vi "卫星模拟器自动控制软件.vi"() -> ()   [LabVIEW 2012]
uses:
  <vilib>/Utility/error.llb/DialogType.ctl
  <vilib>/DAQmx/create/channels.llb/DAQmx Create Channel (DO-Digital Output).vi
  <vilib>/vision/NI_Vision_Development_Module.lvlib
panel:
  in  "缩放比例 (像素/cm)":dbl=4.099468
  in  "远程数据记录器传输状态":bool
  in  "是否下传定位点信息":bool
  in  "远程端口":u16=61557
  in  "本地端口":u16=61556
  in  "远程终端地址":string="localhost"
  in  "broadcast":bool
  in  "是否姿态保持":bool
  out "alpha":dbl
  out "定位点信息":T1(array[cluster]) {"Aspect Ratio" format="%.2f"; "Orientation" format="%.2f"; "Area" format="%.2f"; "Object Center"."Y" format="%.2f"; "Object Center"."X" format="%.2f"}
  in  "Y中心校正":dbl
  in  "X中心校正":dbl
  out "相对偏角(deg)":dbl
  in  "目标Y":dbl
  in  "目标X":dbl
  out "X速率(cm/s)":dbl
  out "Y速率(cm/s)":dbl
  in  "OK Button":bool
  out "角速度(deg/s)":dbl
  in  "气浮状态":bool
  in  "控制频率(Hz)":u32=20
  in  "目标偏角":dbl
  in  "STOP":bool caption="stop (F)"
  out "导航相机输出":T2(plugin-control)
  out "alpha (deg)":dbl
  out "X偏移量 (cm)":dbl
  out "Y偏移量 (cm)":dbl
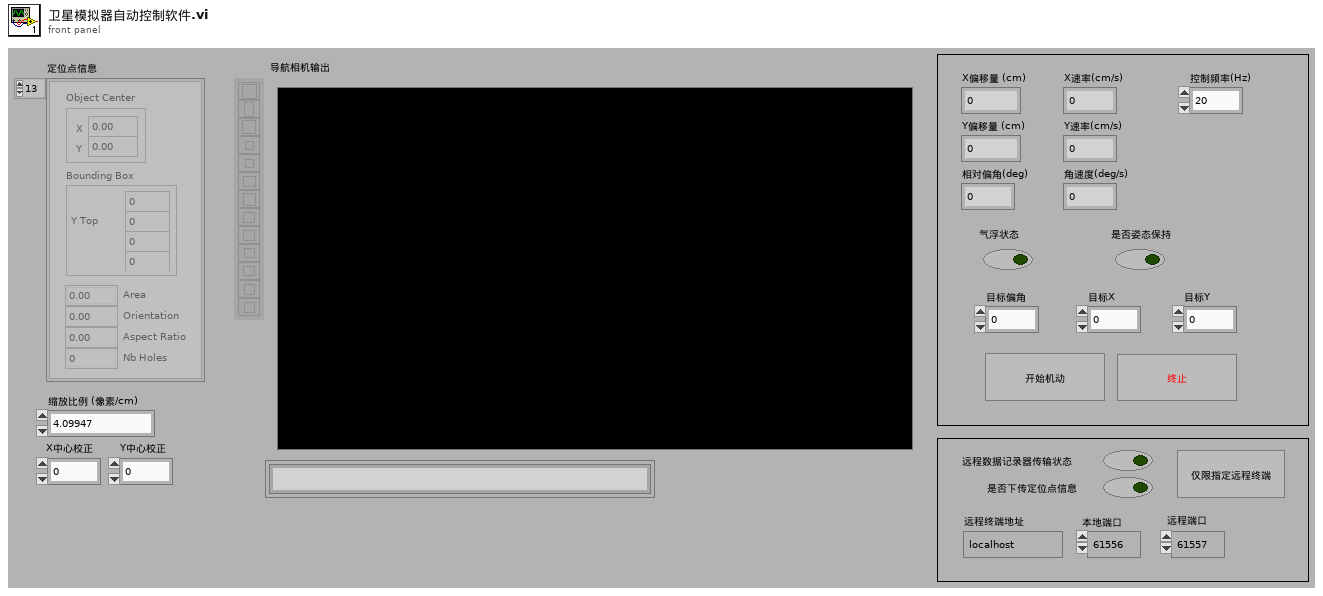
[diagram p1: front panel]
types:
  T1 = cluster{"Object Center":cluster{"X":sgl, "Y":sgl}, "Bounding Box":cluster{"X Left":i32, "Y Top":i32, "X Right":i32, "Y Bottom":i32}, "Area":sgl, "Orientation":sgl, "Aspect Ratio":sgl, "Nb Holes":i32}[]
  T2 = typedef "IMAQ Image.ctl" = refnum<image>
  T3 = typedef "DialogType.ctl" = u16
  T4 = cluster{"X偏移量 (cm)":dbl, "Y偏移量 (cm)":dbl, "相对偏角(deg)":dbl}
  T5 = cluster{"Objects":u16, "Threshold":i32, "Reject Border":bool, "Fill Holes":bool, "Min Object Size":bool, "Min Size":i32, "Max Object Size":bool, "Max Size":i32, "Show Search Area":bool, "Show Center":bool, "Show Bounding Box":bool}
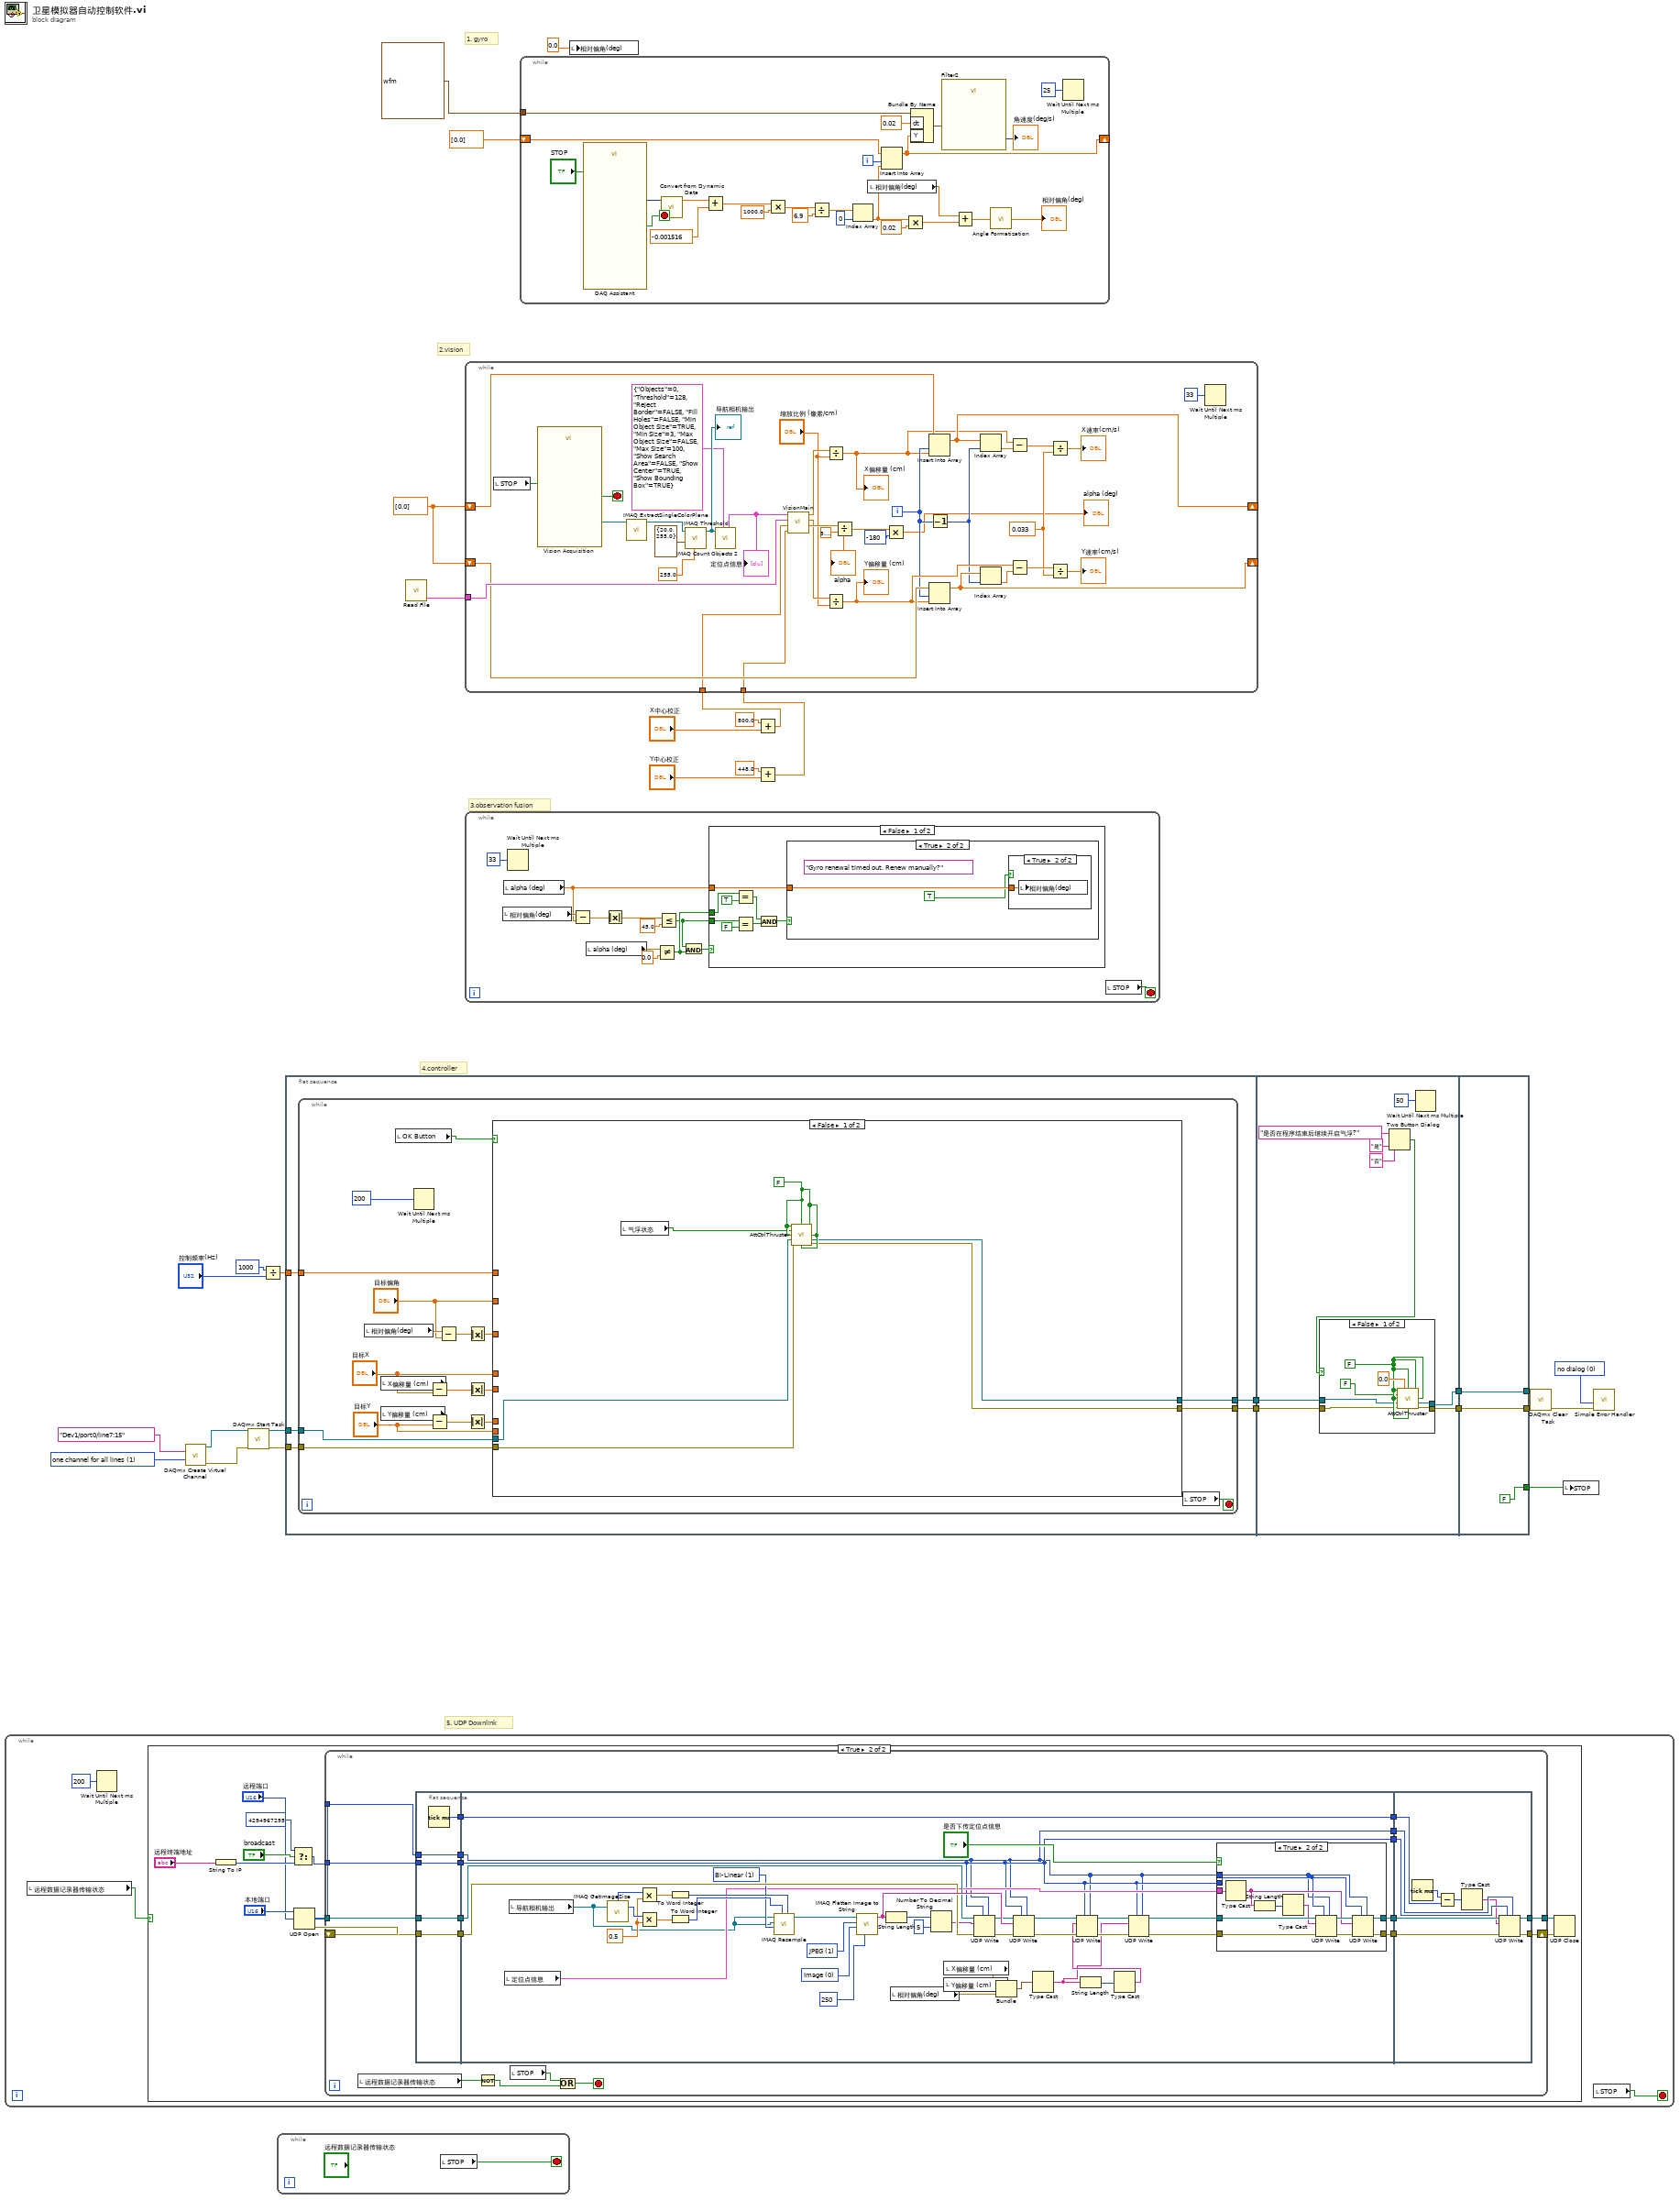
[diagram p0: block diagram]
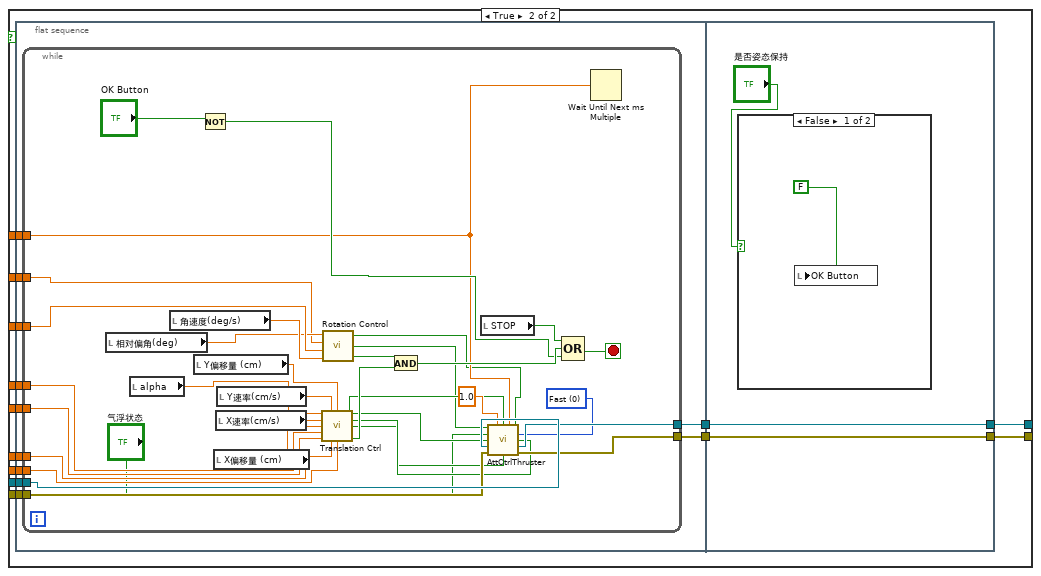
[diagram p4: hidden frame]
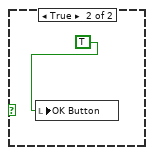
[diagram p5: hidden frame]
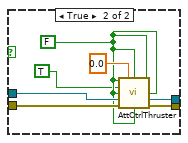
[diagram p6: hidden frame]
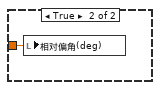
[diagram p9: hidden frame]
diagram:
  w23 = T3 0 items=["no dialog", "OK message", "continue or stop message", "OK message + warnings", "continue/stop + warnings"] ("type of dialog (OK msg:1)")
  w26 = 1 items=["one channel for each line", "one channel for all lines"] ("line grouping")
  w10 = dbl[] [0.0]
  # "5. UDP Downlink"
  # "4.controller"
  # "3.observation fusion"
  # "2.vision"
  # "1. gyro"
  n1 = while {
    stop <- w31 stop-if-true
    n2 = local read "远程数据记录器传输状态"() -> (w32:bool)
    n3 = Wait Until Next ms Multiple(millisecond multiple=u32 200) -> ()  [unwired: 1 out]
    n4 = case shown="True" w32 {
      frame False {
      }
      frame True {
        n5 = String To IP(1:"远程终端地址") -> (0:w40:u32)
        n6 = Select(t=u32 4294967295, s="broadcast", f=w40) -> (s? t:f=w37:u32)
        n7 = UDP Open(11:"本地端口") -> (port=w36:refnum<k16>, 0:w35:errorcluster)  [unwired: 1 in, 4 out]
        n8 = while {
          tunnel: "远程端口" -> [w63]
          tunnel: w37 -> [w62]
          tunnel: w36 -> [w61]
          tunnel: [w59] -> w34
          shift-right: [w58] -> w33
          shift-left: w35 -> [w60]
          stop <- w47 stop-if-true
          n9 = local read "远程数据记录器传输状态"() -> (w45:bool)
          n10 = flat-sequence {
            tunnel: w61 -> [w65]
            tunnel: w63 -> [w66]
            tunnel: w62 -> [w67]
            tunnel: w60 -> [w68]
            tunnel: [w68] -> w57
            tunnel: [w67] -> w56
            tunnel: [w66] -> w55
            tunnel: [w65] -> w54
            tunnel: [w64] -> w53
            tunnel: [w88] -> w52
            tunnel: [w87] -> w51
            tunnel: w57 -> [w106]
            tunnel: w56 -> [w70]
            tunnel: w55 -> [w69]
            tunnel: w54 -> [w90]
            tunnel: [w89] -> w50
            tunnel: w53 -> [w89]
            tunnel: [w69] -> w49
            tunnel: [w70] -> w48
            tunnel: [w130] -> w59
            tunnel: [w124] -> w58
            tunnel: w52 -> [w125]
            tunnel: w51 -> [w131]
            tunnel: w50 -> [w132]
            tunnel: w49 -> [w129]
            tunnel: w48 -> [w128]
            frame #0 {
              n11 = Tick Count (ms)() -> (millisecond timer value=w64:u32)
            }
            frame #1 {
              w94 = u32 1 items=["Zero Order", "Bi-Linear", "Quadratic", "Cubic Spline"] ("Interpolation Type")
              w95 = 0.5
              w103 = 0 items=["Image", "Image and Vision Info", "Reference to Image"] ("Type of Flatten (Image and Vision Info)")
              w108 = 1 items=["None", "JPEG", "PACKED BINARY"] ("Compression (None)")
              n12 = local read "定位点信息"() -> (w85:T1)
              n13 = local read "导航相机输出"() -> (w84:T2)
              n14 = call "IMAQ GetImageSize"("Image"=w84) -> ("Y Resolution"=w96:i32, "X Resolution"=w97:i32)  [unwired: 3 in, 1 out]
              n15 = Multiply(x=w97, y=w95) -> (x*y=w99:dbl)
              n16 = Multiply(x=w96, y=w95) -> (x*y=w101:dbl)
              n17 = To Word Integer(number=w99) -> (16bit integer=w98:i16)
              n18 = To Word Integer(number=w101) -> (16bit integer=w100:i16)
              n19 = call "IMAQ Resample"("X Resolution"=w98, "Y Resolution"=w100, "Interpolation Type"=w94, "Image Dst"=w84, "Image Src"=w84) -> ("Image Dst Out"=w102:T2)  [unwired: 5 in, 1 out]
              n20 = call "IMAQ Flatten Image to String"("Quality (750)"=250, "Type of Flatten (Image and Vision Info)"=w103, "Compression (None)"=w108, "Image"=w102) -> ("Data String"=w107:string)  [unwired: 6 in, 1 out]
              n21 = String Length(string=w107) -> (length=w93:i32)
              n22 = local read "相对偏角(deg)"() -> (w81:dbl)
              n23 = Number To Decimal String(number=w93, width (-)=i16 5) -> (decimal integer string=w92:string)
              n24 = local read "X偏移量 (cm)"() -> (w83:dbl)
              n25 = local read "Y偏移量 (cm)"() -> (w82:dbl)
              n26 = UDP Write(address=w70, port or service name=w69, connection ID=w90, data in=w92, 8:w106) -> (error out=w105:errorcluster, 3:w104:refnum<k16>)  [unwired: 1 out]
              n27 = Bundle("X偏移量 (cm)"=w83, "Y偏移量 (cm)"=w82, "相对偏角(deg)"=w81) -> (w80:T4)  [unwired: 1 in]
              n28 = UDP Write(address=w70, port or service name=w69, connection ID=w104, data in=w107, 8:w105) -> (error out=w78:errorcluster, 3:w79:refnum<k16>)  [unwired: 1 out]
              n29 = Type Cast(x=w80) -> (*(type *) &x=w71:string)  [unwired: 1 in]
              n30 = String Length(string=w71) -> (length=w73:i32)
              n31 = Type Cast(x=w73) -> (*(type *) &x=w72:string)  [unwired: 1 in]
              n32 = UDP Write(address=w70, port or service name=w69, connection ID=w79, data in=w72, 8:w78) -> (error out=w77:errorcluster, 3:w75:refnum<k16>)  [unwired: 1 out]
              n33 = UDP Write(address=w70, port or service name=w69, connection ID=w75, data in=w71, 8:w77) -> (error out=w76:errorcluster, 3:w74:refnum<k16>)  [unwired: 1 out]
              n34 = case shown="True" "是否下传定位点信息" {
                tunnel: w85 -> [_ w123]
                tunnel: w76 -> [w111 w121]
                tunnel: [w111 w119] -> w88
                tunnel: w74 -> [w110 w118]
                tunnel: [w110 w116] -> w87
                tunnel: w70 -> [_ w113]
                tunnel: w69 -> [_ w112]
                frame False {
                }
                frame True {
                  n35 = Type Cast(x=w123) -> (*(type *) &x=w114:string)  [unwired: 1 in]
                  n36 = String Length(string=w114) -> (length=w122:i32)
                  n37 = Type Cast(x=w122) -> (*(type *) &x=w115:string)  [unwired: 1 in]
                  n38 = UDP Write(address=w113, port or service name=w112, connection ID=w118, data in=w115, 8:w121) -> (error out=w120:errorcluster, 3:w117:refnum<k16>)  [unwired: 1 out]
                  n39 = UDP Write(address=w113, port or service name=w112, connection ID=w117, data in=w114, 8:w120) -> (error out=w119:errorcluster, 3:w116:refnum<k16>)  [unwired: 1 out]
                }
              }
            }
            frame #2 {
              n40 = Tick Count (ms)() -> (millisecond timer value=w133:u32)
              n41 = Subtract(x=w133, y=w132) -> (x-y=w127:u32)
              n42 = Type Cast(x=w127) -> (*(type *) &x=w126:string)  [unwired: 1 in]
              n43 = UDP Write(address=w128, port or service name=w129, connection ID=w131, data in=w126, 8:w125) -> (error out=w124:errorcluster, 3:w130:refnum<k16>)  [unwired: 1 out]
            }
          }
          n44 = Not(x=w45) -> (.not. x?=w44:bool)
          n45 = local read "STOP"() -> (w46:bool)
          n46 = Or(x=w46, y=w44) -> (x .or. y?=w47:bool)
        }
        n47 = UDP Close(connection ID=w34, 8:w33) -> ()  [unwired: 2 out]
      }
    }
    n48 = local read "STOP"() -> (w31:bool)
  }
  n49 = call-poly <vilib>:"DAQmx Create Virtual Channel.vi"("lines"=tag "Dev1/port0/line7:15" ("Lines"), "line grouping"=w26) -> ("task out"=w24:refnum<k21>, "error out"=w25:errorcluster)  [unwired: 12 in]
  n50 = call <vilib>:"DAQmx Start Task.vi"("task/channels in"=w24, "error in"=w25) -> ("task out"=w19:refnum<k21>, "error out"=w18:errorcluster)  [unwired: 12 in]
  n51 = Divide(x=u32 1000 ("milliseconds to wait"), y="控制频率(Hz)") -> (x/y=w15:dbl)
  n52 = while {
    stop <- w134 stop-if-true
    n53 = local read "STOP"() -> (w134:bool)
  }
  n54 = flat-sequence {
    tunnel: w19 -> [w139]
    tunnel: w18 -> [w138]
    tunnel: w15 -> [w135]
    tunnel: [w137] -> w14
    tunnel: [w136] -> w13
    tunnel: w14 -> [w237]
    tunnel: w13 -> [w235]
    tunnel: [w236] -> w3
    tunnel: [w234] -> w2
    tunnel: [w253] -> w16
    tunnel: [w254] -> w17
    tunnel: w3 -> [w254]
    tunnel: w2 -> [w253]
    tunnel: [FALSE] -> w1
    frame #0 {
      n55 = while {
        tunnel: w139 -> [w159]
        tunnel: w138 -> [w158]
        tunnel: [w157] -> w137
        tunnel: [w156] -> w136
        tunnel: w135 -> [w141]
        stop <- w155 stop-if-true
        n56 = local read "相对偏角(deg)"() -> (w154:dbl)
        n57 = local read "X偏移量 (cm)"() -> (w150:dbl)
        n58 = local read "Y偏移量 (cm)"() -> (w146:dbl)
        n59 = local read "OK Button"() -> (w142:bool)
        n60 = Wait Until Next ms Multiple(millisecond multiple=200) -> ()  [unwired: 1 out]
        n61 = Subtract(x=w150, y="目标X") -> (x-y=w148:dbl)
        n62 = Subtract(x=w146, y="目标Y") -> (x-y=w144:dbl)
        n63 = Subtract(x=w154, y="目标偏角") -> (x-y=w152:dbl)
        n64 = Absolute Value(x=w152) -> (abs(x)=w151:dbl)
        n65 = Absolute Value(x=w148) -> (abs(x)=w147:dbl)
        n66 = Absolute Value(x=w144) -> (abs(x)=w143:dbl)
        n67 = case shown="False" w142 {
          tunnel: w159 -> [w163 w178]
          tunnel: w158 -> [w162 w177]
          tunnel: [w160 w176] -> w157
          tunnel: [w161 w175] -> w156
          tunnel: w141 -> [_ w174]
          tunnel: "目标偏角" -> [_ w173]
          tunnel: w151 -> [_ w172]
          tunnel: "目标X" -> [_ w171]
          tunnel: w147 -> [_ w170]
          tunnel: "目标Y" -> [_ w169]
          tunnel: w143 -> [_ w168]
          frame False {
            w165 = FALSE
            n68 = local read "气浮状态"() -> (w164:bool)
            n69 = call "AttCtrlThruster.vi"("ctclk"=w165, "Up"=w165, "clkwis"=w165, "Float"=w164, "Left"=w165, "Right"=w165, "task in"=w163, "error in"=w162, "Down"=w165) -> ("task out"=w161:refnum<k21>, "error out"=w160:errorcluster)  [unwired: 5 in]
          }
          frame True {
            n70 = flat-sequence {
              tunnel: w178 -> [w189]
              tunnel: w177 -> [w188]
              tunnel: w174 -> [w185]
              tunnel: w173 -> [w184]
              tunnel: w172 -> [w183]
              tunnel: w171 -> [w182]
              tunnel: w170 -> [w181]
              tunnel: w169 -> [w180]
              tunnel: w168 -> [w179]
              tunnel: [w187] -> w167
              tunnel: [w186] -> w166
              tunnel: [w225] -> w175
              tunnel: [w226] -> w176
              tunnel: w167 -> [w226]
              tunnel: w166 -> [w225]
              frame #0 {
                n71 = while {
                  tunnel: w189 -> [w223]
                  tunnel: w188 -> [w222]
                  tunnel: [w220] -> w187
                  tunnel: [w221] -> w186
                  tunnel: w185 -> [w193]
                  tunnel: w184 -> [w201]
                  tunnel: w183 -> [w216]
                  tunnel: w182 -> [w200]
                  tunnel: w181 -> [w211]
                  tunnel: w180 -> [w199]
                  tunnel: w179 -> [w198]
                  stop <- w217 stop-if-true
                  w207 = u16 0 items=["Fast", "Slow"] ("Angular Acceleration")
                  n72 = local read "相对偏角(deg)"() -> (w214:dbl)
                  n73 = local read "alpha"() -> (w195:dbl)
                  n74 = local read "角速度(deg/s)"() -> (w215:dbl)
                  n75 = local read "Y偏移量 (cm)"() -> (w209:dbl)
                  n76 = Not(x="OK Button") -> (.not. x?=w196:bool)
                  n77 = local read "X偏移量 (cm)"() -> (w212:dbl)
                  n78 = local read "X速率(cm/s)"() -> (w213:dbl)
                  n79 = local read "Y速率(cm/s)"() -> (w210:dbl)
                  n80 = call "Translation Ctrl.vi"("Alpha"=w195, "Filtered Speed Y"=w210, "Y In"=w209, "Filtered Speed X"=w213, "X In"=w212, "X Desired"=w200, "Original Difference X"=w211, "Original Difference Y"=w198, "Y Desired"=w199) -> ("Left"=w205:bool, "Right"=w204:bool, "Down"=w203:bool, "Up"=w202:bool, "Maneuver Complete?"=w206:bool)  [unwired: 2 in]
                  n81 = call "Rotation Control.vi"("Filtered Ohmega"=w215, "Original Difference"=w216, "Alpha Desired"=w201, "Alpha In"=w214) -> ("Maneuver Complete?"=w194:bool, "Counter-ClkWise Rot Ctrl"=w190:bool, "Clockwise Rot Ctrl"=w191:bool)
                  n82 = And(x=w194, y=w206) -> (x .and. y?=w208:bool)
                  n83 = local read "STOP"() -> (w218:bool)
                  n84 = call "AttCtrlThruster.vi"("ctclk"=w190, "Duty Cycle"=1.0, "Up"=w202, "Period"=w193, "clkwis"=w191, "Float"="气浮状态", "Angular Acceleration"=w207, "Left"=w205, "Right"=w204, "task in"=w223, "error in"=w222, "Down"=w203) -> ("task out"=w221:refnum<k21>, "error out"=w220:errorcluster)  [unwired: 2 in]
                  n85 = Compound Arithmetic op=OR(w218, w208, w196) -> (w217:bool)
                  n86 = Wait Until Next ms Multiple(millisecond multiple=w193) -> ()  [unwired: 1 out]
                }
              }
              frame #1 {
                n87 = case shown="False" "是否姿态保持" {
                  frame False {
                    n88 = local write "OK Button"(FALSE) -> ()
                  }
                  frame True {
                    n89 = local write "OK Button"(TRUE) -> ()
                  }
                }
              }
            }
          }
        }
        n90 = local read "STOP"() -> (w155:bool)
      }
    }
    frame #1 {
      n91 = Two Button Dialog(message="是否在程序结束后继续开启气浮?", 1:"否" ("F button name (\"Cancel\")"), 2:"是" ("T button name (\"OK\")")) -> (T button?=w231:bool)
      n92 = case shown="False" w231 {
        tunnel: w237 -> [w240 w251]
        tunnel: [w238 w250] -> w236
        tunnel: w235 -> [w241 w249]
        tunnel: [w239 w248] -> w234
        frame False {
          w243 = FALSE
          n93 = call "AttCtrlThruster.vi"("ctclk"=w243, "Duty Cycle"=0.0, "Up"=w243, "clkwis"=w243, "Float"=FALSE, "Left"=w243, "Right"=w243, "task in"=w241, "error in"=w240, "Down"=w243) -> ("task out"=w239:refnum<k21>, "error out"=w238:errorcluster)  [unwired: 4 in]
        }
        frame True {
          w246 = FALSE
          n94 = call "AttCtrlThruster.vi"("ctclk"=w246, "Duty Cycle"=0.0, "Up"=w246, "clkwis"=w246, "Float"=TRUE, "Left"=w246, "Right"=w246, "task in"=w249, "error in"=w251, "Down"=w246) -> ("task out"=w248:refnum<k21>, "error out"=w250:errorcluster)  [unwired: 4 in]
        }
      }
      n95 = Wait Until Next ms Multiple(millisecond multiple=u32 50) -> ()  [unwired: 1 out]
    }
    frame #2 {
    }
  }
  n96 = call "Read File.vi"() -> ("Objects"=w29:T1)  [unwired: 1 in, 1 out]
  n97 = while {
    stop <- w265 stop-if-true
    n98 = local read "相对偏角(deg)"() -> (w264:dbl)
    n99 = local read "alpha (deg)"() -> (w260:dbl)
    n100 = Wait Until Next ms Multiple(millisecond multiple=u32 33) -> ()  [unwired: 1 out]
    n101 = Subtract(x=w264, y=w260) -> (x-y=w263:dbl)
    n102 = local read "alpha (deg)"() -> (w258:dbl)
    n103 = Absolute Value(x=w263) -> (abs(x)=w262:dbl)
    n104 = Not Equal?(x=w258, y=0.0) -> (x != y?=w256:bool)
    n105 = Less Or Equal?(x=w262, y=45.0) -> (x <= y?=w255:bool)
    n106 = And(x=w255, y=w256) -> (x .and. y?=w259:bool)
    n107 = case shown="False" w259 {
      tunnel: w260 -> [w267 w278]
      tunnel: w256 -> [w269 _]
      tunnel: w255 -> [w268 _]
      frame False {
        n108 = Equal?(x=w269, y=TRUE) -> (x = y?=w273:bool)
        n109 = Equal?(x=w268, y=FALSE) -> (x = y?=w272:bool)
        n110 = And(x=w273, y=w272) -> (x .and. y?=w270:bool)
        n111 = case shown="True" w270 {
          tunnel: w267 -> [_ w276]
          frame False {
          }
          frame True {
            (unwired) "Gyro renewal timed out. Renew manually?" ("message")
            n112 = case shown="True" TRUE {
              tunnel: w276 -> [_ w277]
              frame False {
              }
              frame True {
                n113 = local write "相对偏角(deg)"(w277) -> ()
              }
            }
          }
        }
      }
      frame True {
        n114 = local write "相对偏角(deg)"(w278) -> ()
      }
    }
    n115 = local read "STOP"() -> (w265:bool)
  }
  n116 = while {
    shift-right: [w286] -> _
    shift-left: dbl[] [0.0] -> [w287]
    tunnel: waveform(dbl) {"t0"=timestamp(0 s since 1904-01-01), "dt"=1.0, "Y"=[]} ("waveform") -> [w284]
    i -> [w285]
    stop <- w302 stop-if-true
    n117 = call "DAQ Assistant"("stop (F)"="STOP") -> ("data"=w294:dynamicdata, "stopped"=w302:bool)  [unwired: 15 in, 2 out]
    n118 = call "Convert from Dynamic Data"("Dynamic Data Type"=w294) -> ("Array"=w292:dbl[])  [unwired: 3 in]
    n119 = Add(x=w292, y=-0.001516) -> (x+y=w290:dbl[])
    n120 = Multiply(x=w290, y=1000.0) -> (x*y=w301:dbl[])
    n121 = Divide(x=w301, y=6.9) -> (x/y=w295:dbl[])
    n122 = Index Array(array=w295, index=0) -> (element=w280:dbl)
    n123 = local read "相对偏角(deg)"() -> (w289:dbl)
    n124 = Insert Into Array(array=w287, index=w285, new element=w280) -> (w286:dbl[])
    n125 = Multiply(x=w280, y=0.02) -> (x*y=w296:dbl)
    n126 = Bundle By Name(cluster=w284, "dt"=0.02, "Y"=w286) -> (w283:waveform(dbl))
    n127 = call "Filter2"("Signal"=w283) -> ("Filtered Signal"=→"角速度(deg/s)":dynamicdata)  [unwired: 9 in, 1 out]
    n128 = Add(x=w289, y=w296) -> (x+y=w282:dbl)
    n129 = call "Angle Formatization.vi"("Alpha"=w282) -> ("Alpha Formatized"=→"相对偏角(deg)":dbl)
    n130 = Wait Until Next ms Multiple(millisecond multiple=u32 25 ("y")) -> ()  [unwired: 1 out]
  }
  n131 = local write "相对偏角(deg)"(0.0 ("y")) -> ()
  n132 = Add(x=800.0 ("c_x"), y="X中心校正") -> (x+y=w7:dbl)
  n133 = Add(x=448.0 ("c_y"), y="Y中心校正") -> (x+y=w4:dbl)
  n134 = while {
    tunnel: w29 -> [w328]
    shift-right: [w325] -> _
    shift-left: w10 -> [w326]
    shift-right: [w314] -> _
    shift-left: w10 -> [w317]
    tunnel: w4 -> [w307]
    tunnel: w7 -> [w306]
    i -> [w316]
    stop <- w339 stop-if-true
    w310 = 0.033 ("y")
    n135 = local read "STOP"() -> (w330:bool)
    n136 = call "Vision Acquisition"("Stop (F)"=w330) -> ("Image Out"=w334:T2, "Stopped"=w339:bool)  [unwired: 24 in, 1 out]
    n137 = call "IMAQ ExtractSingleColorPlane"("Image Src"=w334) -> ("Image Dst Out"=w338:T2)  [unwired: 9 in, 1 out]
    n138 = call "IMAQ Threshold"("Replace Value"=sgl 255.0 ("replace value"), "Range"=cluster{"lower value":sgl, "upper value":sgl} {"lower value"=20.0, "upper value"=255.0} ("threshold"), "Image Src"=w338) -> ("Image Dst Out"=w335:T2)  [unwired: 7 in, 1 out]
    "导航相机输出" <- w335
    n139 = call "IMAQ Count Objects 2"("Settings"=T5 {"Objects"=0, "Threshold"=128, "Reject Border"=FALSE, "Fill Holes"=FALSE, "Min Object Size"=TRUE, "Min Size"=3, "Max Object Size"=FALSE, "Max Size"=100, "Show Search Area"=FALSE, "Show Center"=TRUE, "Show Bounding Box"=TRUE}, "Image"=w335) -> ("Objects"=w329:T1)  [unwired: 5 in, 4 out]
    "定位点信息" <- w329
    n140 = call "VisionMain.vi"("Y Center"=w307, "X Center"=w306, "Original Plots"=w328, "Plots Captured"=w329) -> ("alpha"=w327:dbl, "dy"=w323:dbl, "dx"=w318:dbl)  [unwired: 5 in]
    "alpha" <- w327
    n141 = Divide(x=w318, y="缩放比例 (像素/cm)") -> (x/y=w313:dbl)
    "X偏移量 (cm)" <- w313
    n142 = Divide(x=w323, y="缩放比例 (像素/cm)") -> (x/y=w322:dbl)
    "Y偏移量 (cm)" <- w322
    n143 = Divide(x=w327, y=3.141592653589793) -> (x/y=w332:dbl)
    n144 = Multiply(x=w332, y=-180) -> (x*y=→"alpha (deg)":dbl)
    n145 = Insert Into Array(array=w317, index=w316, new element=w313) -> (w314:dbl[])
    n146 = Insert Into Array(array=w326, index=w316, new element=w322) -> (w325:dbl[])
    n147 = Decrement(x=w316) -> (x-1=w315:i32)
    n148 = Index Array(array=w314, index=w315) -> (element=w312:dbl)
    n149 = Index Array(array=w325, index=w315) -> (element=w324:dbl)
    n150 = Subtract(x=w313, y=w312) -> (x-y=w311:dbl)
    n151 = Subtract(x=w322, y=w324) -> (x-y=w321:dbl)
    n152 = Divide(x=w311, y=w310) -> (x/y=→"X速率(cm/s)":dbl)
    n153 = Divide(x=w321, y=w310) -> (x/y=→"Y速率(cm/s)":dbl)
    n154 = Wait Until Next ms Multiple(millisecond multiple=u32 33) -> ()  [unwired: 1 out]
  }
  n155 = call <vilib>:"DAQmx Clear Task.vi"("task in"=w16, "error in"=w17) -> ("error out"=w22:errorcluster)  [unwired: 13 in]
  n156 = local write "STOP"(w1) -> ()
  n157 = call <vilib>:"Simple Error Handler.vi"("type of dialog (OK msg:1)"=w23, "error in (no error)"=w22) -> ()  [unwired: 3 in, 5 out]
